vi "DI Read_TS.vi"(8 "error in (no error)":errorcluster) -> (0 "error out":errorcluster, 1 "DI Reading (Hex String)":string, 2 "DI Reading":bool[](array[boolean]), 3 "VISA Refnum out":refnum<visa-resource-name>)   [LabVIEW 2022 SP3]
uses:
  <vilib>/Instr/_visa.llb/VISA Flush IO Buffer Mask.ctl
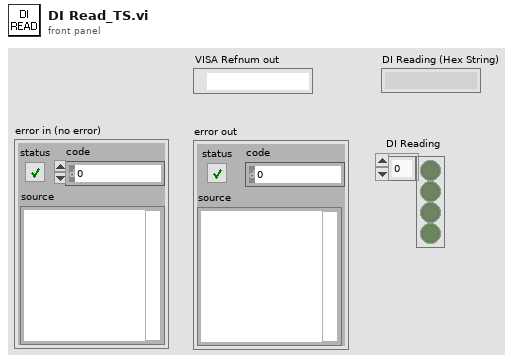
[diagram p1: front panel]
types:
  T1 = typedef "VISA Flush IO Buffer Mask.ctl" = u16
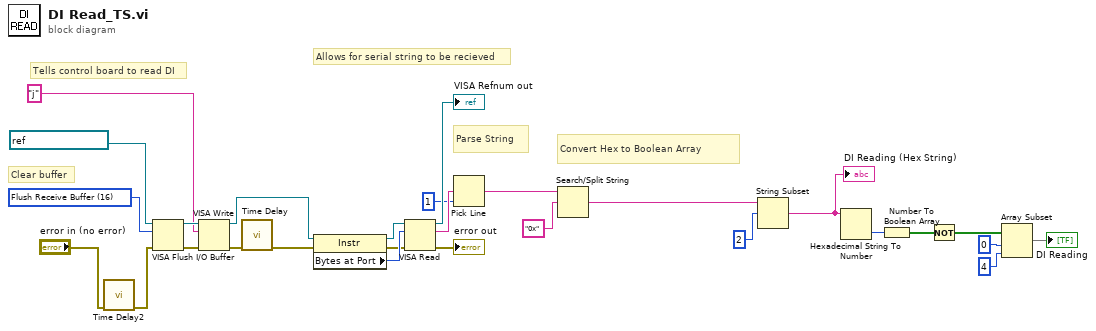
[diagram p0: block diagram]
diagram:
  w17 = T1 16 items=["Flush Receive Buffer"=16, "Write Transmit Buffer to Device"=32, "Flush Receive Buffer (No I/O)"=64, "Flush Transmit Buffer"=128] ("Mask")
  # "Convert Hex to Boolean Array"
  # "Clear buffer"
  # "Parse String"
  # "Allows for serial string to be recieved"
  # "Tells control board to read DI"
  n1 = call "Time Delay2"("error in (no error)"="error in (no error)") -> ("error out"=w3:errorcluster)  [unwired: 10 in]
  n2 = VISA Flush I/O Buffer(VISA resource name=refnum<visa-resource-name> "ControlBoard", mask (16)=w17, error in (no error)=w3) -> (VISA resource name out=w19:refnum<visa-resource-name>, error out=w20:errorcluster)
  n3 = VISA Write(VISA resource name=w19, write buffer="j", error in (no error)=w20) -> (VISA resource name out=w22:refnum<visa-resource-name>, error out=w18:errorcluster)  [unwired: 1 out]
  n4 = call "Time Delay"("error in (no error)"=w18) -> ("error out"=w21:errorcluster)  [unwired: 10 in]
  n5 = property class="Instr"(reference=w22, error in=w21) -> (reference out=w14:refnum<visa-resource-name>, error out=w15:errorcluster, "Bytes at Port"=w16:u32)
  n6 = VISA Read(VISA resource name=w14, byte count=w16, error in (no error)=w15) -> (VISA resource name out=→"VISA Refnum out":refnum<visa-resource-name>, read buffer=w26:string, error out=→"error out":errorcluster)  [unwired: 1 out]
  n7 = Pick Line(multi-line string=w26, line index=1) -> (output string=w27:string)  [unwired: 1 in]
  n8 = Search/Split String(string=w27, search string/char (-)="0x" ("regular expression")) -> (match + rest of string=w24:string)  [unwired: 1 in, 2 out]
  n9 = String Subset(string=w24, offset (0)=2) -> (substring=w8:string)  [unwired: 1 in]
  "DI Reading (Hex String)" <- w8
  n10 = Hexadecimal String To Number(string=w8) -> (number=w10:u32)  [unwired: 2 in, 1 out]
  n11 = Number To Boolean Array(number=w10) -> (Boolean array=w9:bool[])
  n12 = Not(x=w9) -> (.not. x?=w5:bool[])
  n13 = Array Subset(array=w5, index=0, length=4) -> (→"DI Reading":bool[])
